vi "Freeze CMD PID.vi"(0 "Output In":dbl format="%#_13g", 7 "FreezeCmdPID":bool, 11 "Step":dbl format="%#_13g") -> (4 "Output Out":dbl format="%#_13g")   [LabVIEW 2019]
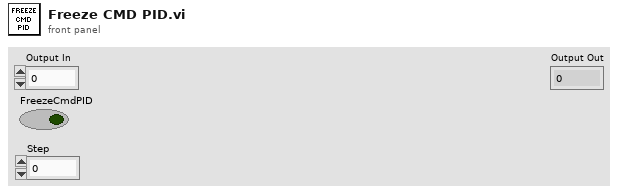
[diagram p1: front panel]
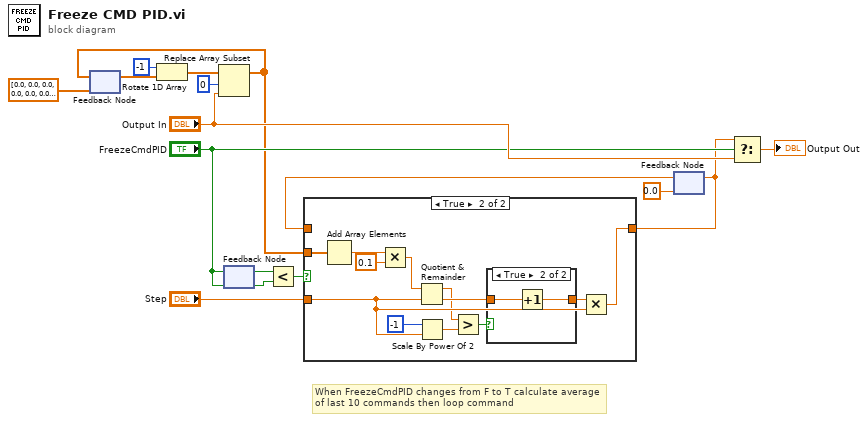
[diagram p0: block diagram]
diagram:
  # "When FreezeCmdPID changes from F to T calculate average\nof last 10 commands then loop command"
  n1 = feedback #1(dbl[] [0.0, 0.0, 0.0, 0.0, 0.0, 0.0, 0.0, 0.0, 0.0, 0.0]) -> (w13:dbl[])
  n2 = Rotate 1D Array(1:w13, 2:-1 ("n")) -> (0:w15:dbl[])
  n3 = Replace Array Subset(array=w15, new element="Output In", index=0) -> (w4:dbl[])
  n4 = feedback-in #1(w4) -> ()
  n5 = feedback-in #2("FreezeCmdPID") -> ()
  n6 = feedback #2("FreezeCmdPID") -> (w6:bool)
  n7 = Less?(x=w6, y="FreezeCmdPID") -> (x < y?=w5:bool)
  n8 = feedback #3(0.0) -> (w2:dbl)
  n9 = case shown="True" w5 {
    tunnel: "Step" -> [_ w28]
    tunnel: w4 -> [_ w20]
    tunnel: [w16 w18] -> w1
    tunnel: w2 -> [w16 _]
    frame False {
    }
    frame True {
      n10 = Add Array Elements(numeric array=w20) -> (sum=w21:dbl)
      n11 = Multiply(x=w21, y=0.1) -> (x*y=w19:dbl)
      n12 = Quotient & Remainder(x=w19, y=w28) -> (x-y*floor(x/y)=w17:dbl, floor(x/y)=w24:dbl)
      n13 = Scale By Power Of 2(n=i16 -1, x=w28) -> (x*2^n=w26:dbl)
      n14 = Greater?(x=w17, y=w26) -> (0:w25:bool)
      n15 = case shown="True" w25 {
        tunnel: w24 -> [w29 w31]
        tunnel: [w29 w30] -> w23
        frame False {
        }
        frame True {
          n16 = Increment(x=w31) -> (x+1=w30:dbl)
        }
      }
      n17 = Multiply(x=w23, y=w28) -> (x*y=w18:dbl)
    }
  }
  n18 = feedback-in #3(w1) -> ()
  n19 = Select(t=w1, s="FreezeCmdPID", f="Output In") -> (s? t:f=→"Output Out":dbl)
